vi "Broadcast Message.vi"(8 "error in (no error)":errorcluster, 9 "Message Data":variant, 10 "Message":string, 11 "Asynchronous Action In":refnum<class "Async Action.lvclass">) -> (0 "error out":errorcluster, 3 "Asynchronous Action Out":refnum<class "Async Action.lvclass">)   [LabVIEW 2020, in "Async Action.lvclass"]
doc: "Method for broadcasting the state of the helper loop. The framework will send messages when it is started and stopped."
uses:
  Async Action.lvclass
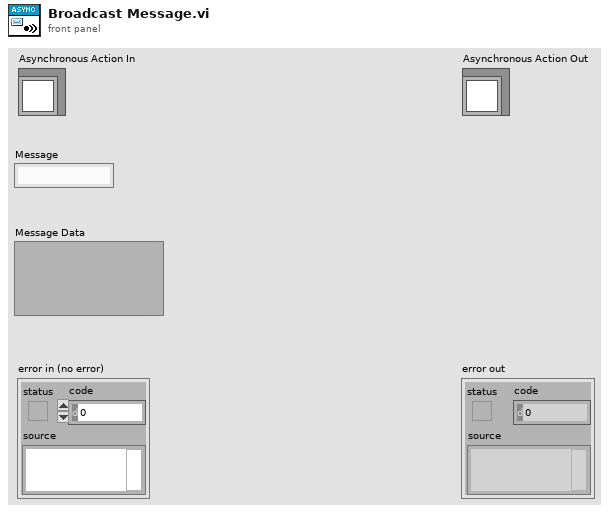
[diagram p1: front panel]
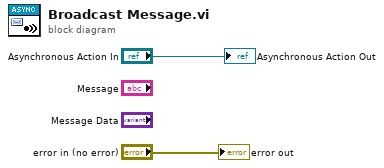
[diagram p0: block diagram]
diagram:
  "error out" <- "error in (no error)"
  "Asynchronous Action Out" <- "Asynchronous Action In"
